vi "Make pulse signal.vi"(6 "cyclesperpulse":dbl=10.0 caption="Cycles per pulse", 7 "Output freq (Hz)":dbl=50.0, 8 "sinamp":dbl=20.0 caption="sineamp", 9 "sinfreq":dbl=1.5 caption="sinefreq", 10 "total time":dbl=20.0, 11 "pulse data":T2) -> (1 "phases":T1, 2 "pulse signal":dbl[](array[numeric]), 3 "sine signal":dbl[](array[numeric]))   [LabVIEW 2013]
uses:
  Pulse data.ctl
  Phases.ctl
  <vilib>/Analysis/1siggen.llb/Ramp Pattern by Samples.vi
  <vilib>/Analysis/1siggen.llb/General Aperiodic Triangle.vi
  <vilib>/Analysis/NI_AALBase.lvlib
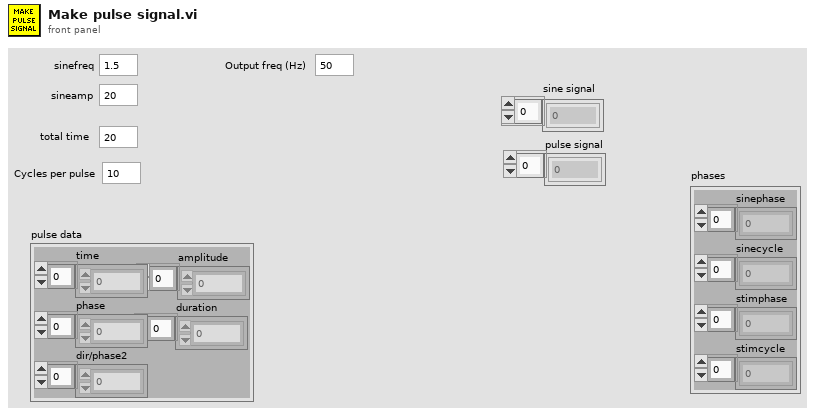
[diagram p1: front panel]
types:
  T1 = typedef "Phases.ctl" = cluster{"sinephase":dbl[], "sinecycle":dbl[], "stimphase":dbl[], "stimcycle":dbl[]}
  T2 = typedef "Pulse data.ctl" = cluster{"time":dbl[], "phase":dbl[], "dir/phase2":dbl[], "amplitude":dbl[], "duration":dbl[]}
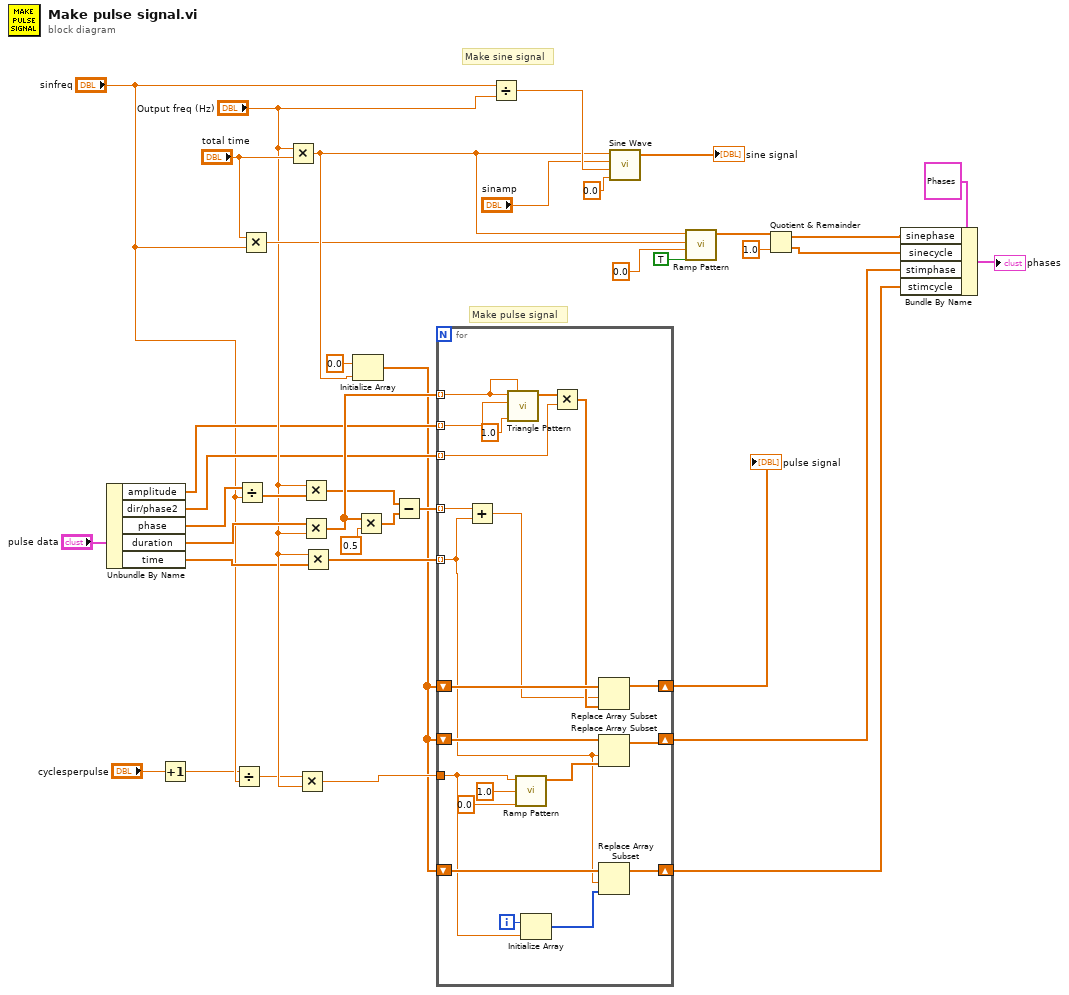
[diagram p0: block diagram]
diagram:
  # "Make pulse signal"
  # "Make sine signal"
  n1 = Unbundle By Name("pulse data") -> ("amplitude"=w14:dbl[], "dir/phase2"=w15:dbl[], "phase"=w22:dbl[], "duration"=w35:dbl[], "time"=w18:dbl[])
  n2 = Increment(x="cyclesperpulse") -> (x+1=w1:dbl)
  n3 = Divide(x=w1, y="sinfreq") -> (x/y=w3:dbl)
  n4 = Divide(x=w22, y="sinfreq") -> (x/y=w21:dbl[])
  n5 = Multiply(x="total time", y="sinfreq") -> (x*y=w25:dbl)
  n6 = Multiply(x="Output freq (Hz)", y="total time") -> (x*y=w29:dbl)
  n7 = Multiply(x=w3, y="Output freq (Hz)") -> (x*y=w16:dbl)
  n8 = Multiply(x="Output freq (Hz)", y=w21) -> (x*y=w19:dbl[])
  n9 = Multiply(x=w35, y="Output freq (Hz)") -> (x*y=w33:dbl[])
  n10 = Multiply(x="Output freq (Hz)", y=w18) -> (x*y=w17:dbl[])
  n11 = Initialize Array(0.0 ("element"), w29) -> (w13:dbl[])
  n12 = Multiply(x=w33, y=0.5) -> (x*y=w31:dbl[])
  n13 = Subtract(x=w19, y=w31) -> (x-y=w30:dbl[])
  n14 = for {
    tunnel: w33 -> [w59] mode=indexing
    tunnel: w14 -> [w60] mode=indexing
    tunnel: w30 -> [w49] mode=indexing
    tunnel: w15 -> [w56] mode=indexing
    shift-right: [w53] -> w10
    shift-left: w13 -> [w55]
    shift-right: [w46] -> w6
    shift-left: w13 -> [w47]
    tunnel: w17 -> [w40] mode=indexing
    tunnel: w16 -> [w41]
    shift-right: [w42] -> w5
    shift-left: w13 -> [w44]
    i -> [w50]
    n15 = Add(x=w49, y=w40) -> (x+y=w48:dbl)
    n16 = call <vilib>:"Triangle Pattern.vi"("width (s)"=w59, "delta t (s)"=1.0, "amplitude"=w60, "samples"=w59) -> ("Triangle Pattern"=w57:dbl[])  [unwired: 6 in, 1 out]
    n17 = call-poly <vilib>:"Ramp Pattern.vi"("start"=0.0, "end"=1.0, "samples"=w41) -> ("Ramp Pattern"=w45:dbl[])  [unwired: 7 in, 1 out]
    n18 = Initialize Array(w50, w41) -> (w43:i32[])
    n19 = Multiply(x=w57, y=w56) -> (x*y=w54:dbl[])
    n20 = Replace Array Subset(array=w55, new element=w54, index=w48) -> (w53:dbl[])
    n21 = Replace Array Subset(array=w47, new element=w45, index=w40) -> (w46:dbl[])
    n22 = Replace Array Subset(array=w44, new element=w43, index=w40) -> (w42:dbl[])
  }
  "pulse signal" <- w10
  n23 = Divide(x="sinfreq", y="Output freq (Hz)") -> (x/y=w39:dbl)
  n24 = call <vilib>:"Sine Wave.vi"("samples"=w29, "amplitude"="sinamp", "frequency"=w39, "phase in"=0.0) -> ("sine wave"=→"sine signal":dbl[])  [unwired: 1 in, 2 out]
  n25 = call-poly <vilib>:"Ramp Pattern.vi"("exclude end?"=TRUE, "start"=0.0, "end"=w25, "samples"=w29) -> ("Ramp Pattern"=w28:dbl[])  [unwired: 6 in, 1 out]
  n26 = Quotient & Remainder(x=w28, y=1.0 ("start")) -> (x-y*floor(x/y)=w8:dbl[], floor(x/y)=w7:dbl[])
  n27 = Bundle By Name(cluster=T1 {"sinephase"=array[5367 elements], "sinecycle"=array[5367 elements], "stimphase"=array[5367 elements], "stimcycle"=array[5367 elements]} ("phases"), "sinephase"=w8, "sinecycle"=w7, "stimphase"=w6, "stimcycle"=w5) -> (→"phases":T1)
